vi "MakeBar-ADC.vi"() -> (0 "output array":u8[](array[numeric]), 1 "Input Spectrum":dynamicdata(graph))   [LabVIEW 2018]
uses:
  <vilib>/express/express analysis/Spectral/Block/exnSpectralBlock spectral measurements RMS poly.vi
  <vilib>/express/express analysis/Spectral/Block/exnSpectralBlock spectral measurements RMS DDT.vi
  <vilib>/express/express analysis/Spectral/XNode/ExpressSpectralMeasurementsBlockNode.xnode
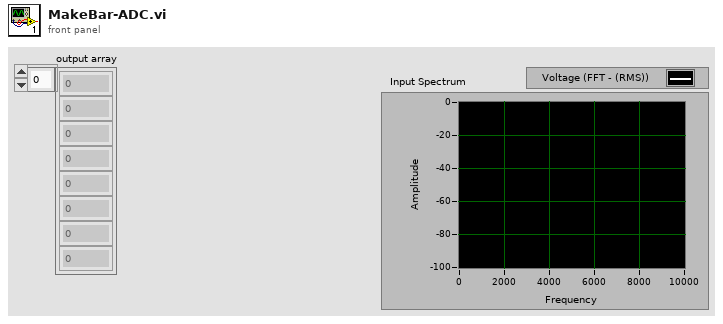
[diagram p1: front panel]
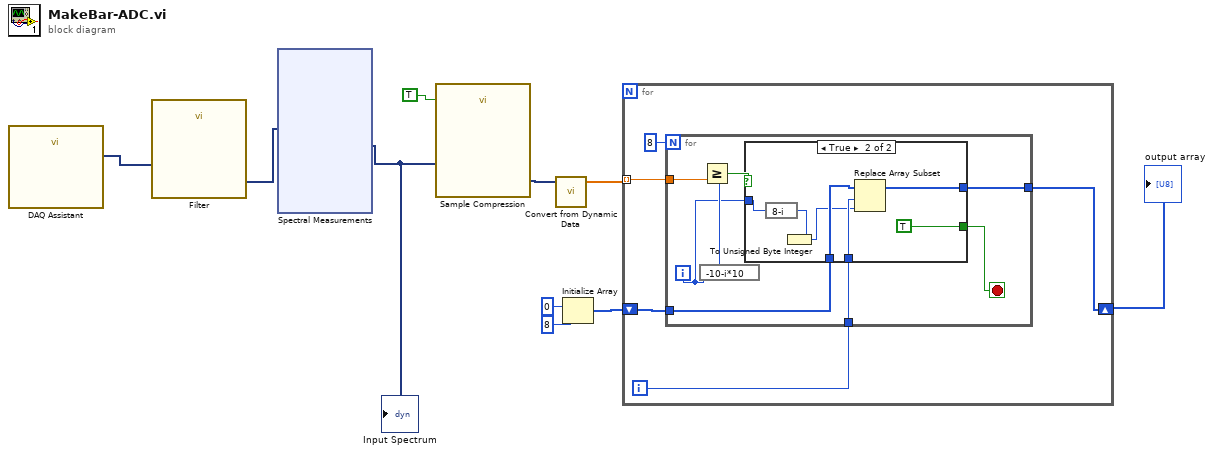
[diagram p0: block diagram]
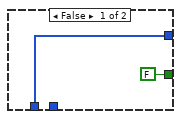
[diagram p2: hidden frame]
diagram:
  n1 = call "DAQ Assistant"() -> ("data"=w2:dynamicdata)  [unwired: 17 in, 2 out]
  n2 = call "Filter"("Signal"=w2) -> ("Filtered Signal"=w1:dynamicdata)  [unwired: 9 in, 1 out]
  n3 = xnode "Spectral Measurements"("Signals"=w1) -> ("FFT - (RMS)"=w5:dynamicdata)  [unwired: 1 in, 2 out]
  "Input Spectrum" <- w5
  n4 = call "Sample Compression"("Enable"=TRUE, "Signals"=w5) -> ("Maximum"=w4:dynamicdata)  [unwired: 7 in, 2 out]
  n5 = call "Convert from Dynamic Data"("Dynamic Data Type"=w4) -> ("Array"=w3:dbl[])  [unwired: 3 in]
  n6 = Initialize Array(u8 0 ("element"), 8 ("dimension size")) -> (w7:u8[])
  n7 = for {
    tunnel: w3 -> [w14] mode=indexing
    shift-right: [w11] -> w6
    shift-left: w7 -> [w12]
    i -> [w13]
    n8 = for {
      N: 8 -> [_]
      tunnel: w14 -> [w22]
      tunnel: w13 -> [w20]
      tunnel: w12 -> [w18]
      tunnel: [w19] -> w11
      i -> [w21]
      stop <- w16 stop-if-true
      n9 = expression code="-10-i*10"(w21) -> (w23:i32)
      n10 = Greater Or Equal?(x=w22, y=w23) -> (x >= y?=w17:bool)
      n11 = case shown="True" w17 {
        tunnel: w21 -> [_ w31]
        tunnel: w20 -> [_ w32]
        tunnel: w18 -> [w25 w30]
        tunnel: [w25 w27] -> w19
        tunnel: [FALSE TRUE] -> w16
        frame False {
        }
        frame True {
          n12 = expression code="8-i"(w31) -> (w29:i32)
          n13 = To Unsigned Byte Integer(number=w29) -> (unsigned 8bit integer=w28:u8)
          n14 = Replace Array Subset(array=w30, new element=w28, index=w32) -> (w27:u8[])
        }
      }
    }
  }
  "output array" <- w6
